vi "Measure vs B2Dv4.vi"() -> ()   [LabVIEW 2009]
doc: "This VI is an example operator panel.\n\nThe VI contains a table for the field values that may be configured manually, or loaded by checking the \"Prompt for File\" box. The data file should contain 3 columns of data, with each column delimited by a tab character.\n\nBefore the VI is executed, set the desired field units and coordinate system. Once the VI is started, follow the directions in the STATUS indicator to operate. Once a field value is achieved, it will be held indefinitely with no user intervention.\n\nThe present field is displayed in the selected units and coordinate system. The present field is queried once per second.\n\nIf a field point is specified that is outside the limits for the magnet, the VI will abort execution."
uses:
  <vilib>/Utility/file.llb/Read From Spreadsheet File (DBL).vi
panel:
  in  "Wait between \nVectors":bool
  in  "FieldRange":dbl=1.0
  in  "Change\nPID\n(DetermineSIMPID.vi)":bool
  in  "Wait between \nVectors (ms)":u32=3000
  in  "X Axis":enum16{"B", "phi"}(ring)
  in  "Y Axis":T1(ring)=enum."HP (V)"
  out "measured data":dbl[][](array[numeric])=[[1.000012086526958, 89.00072302371139, 0.0, 0.0, 0.0, 0.0, 0.0, 0.0, 0.0, 0.0, 20.70647, 3397102510.2661195], [0.9999822655427446, 89.00012016557346, 0.0, 0.0, 0.0, 0.0, 0.0, 0.0, 0.0, 0.0, 20.70772, 3397102511.0341196], [1.0000224339983579, 88.99958730013925, 0.0, 0.0, 0.0, 0.0, 0.0, 0.0, 0.0, 0.0, 20.70752, 3397102511.6071196], [1.0000220850061263, 89.00073301575388, 0.0, 0.0, 0.0, 0.0, 0.0, 0.0, 0.0, 0.0, 20.70772, 3397102512.18112], [0.9999922640200775, 89.00013016394165, 0.0, 0.0, 0.0, 0.0, 0.0, 0.0, 0.0, 0.0, 20.70689, 3397102512.7561197], [1.0000022624974407, 89.0001401621099, 0.0, 0.0, 0.0, 0.0, 0.0, 0.0, 0.0, 0.0, 20.70783, 3397102513.3311195], [1.0000122609748343, 89.00015016007822, 0.0, 0.0, 0.0, 0.0, 0.0, 0.0, 0.0, 0.0, 20.70835, 3397102513.9071198], [1.00000208804782, 89.00071303146908, 0.0, 0.0, 0.0, 0.0, 0.0, 0.0, 0.0, 0.0, 20.70845, 3397102514.4801197], [0.9999822655427446, 89.00012016557346, 0.0, 0.0, 0.0, 0.0, 0.0, 0.0, 0.0, 0.0, 20.70793, 3397102515.05712], [1.0000122609748343, 89.00015016007822, 0.0, 0.0, 0.0, 0.0, 0.0, 0.0, 0.0, 0.0, 20.70731, 3397102515.63012], [1.0000022624974407, 89.0001401621099, 0.0, 0.0, 0.0, 0.0, 0.0, 0.0, 0.0, 0.0, 20.70731, 3397102516.2041197], [0.9999822655427446, 89.00012016557346, 0.0, 0.0, 0.0, 0.0, 0.0, 0.0, 0.0, 0.0, 20.70606, 3397102516.7781196], [0.9999822655427446, 89.00012016557346, 0.0, 0.0, 0.0, 0.0, 0.0, 0.0, 0.0, 0.0, 20.70595, 3397102517.46612], [1.0000122609748343, 89.00015016007822, 0.0, 0.0, 0.0, 0.0, 0.0, 0.0, 0.0, 0.0, 20.70595, 3397102518.03712], [0.9999724416202679, 88.9995372806674, 0.0, 0.0, 0.0, 0.0, 0.0, 0.0, 0.0, 0.0, 20.70606, 3397102518.6131196]]
  out "XY Graph":T2(graph)={"measured data"=[1.000012086526958, 0.9999822655427446, 1.0000224339983579, 1.0000220850061263, 0.9999922640200775, 1.0000022624974407, 1.0000122609748343, 1.00000208804782, 0.9999822655427446, 1.0000122609748343, 1.0000022624974407, 0.9999822655427446, 0.9999822655427446, 1.0000122609748343, 0.9999724416202679], "measured data"=[20.70647, 20.70772, 20.70752, 20.70772, 20.70689, 20.70783, 20.70835, 20.70845, 20.70793, 20.70731, 20.70731, 20.70606, 20.70595, 20.70595, 20.70606]}
  in  "Notes:":string="Datum: 24.08.11, Uhrzeit: 16:26, T0.3K, PID LOOP: P -0.2 I 200 D off , PID Dämpfung: P off , Laser 25°, 20mA, AOM 10mA, Sweep 0.12T/min, Winkelsweep 90-0--280° bei 1 T,  Winkelschritt 0.4°, Position auf ansteigender Fringe" caption="Notizen:"
  out "Messfile Refnum":refnum<file>
  in  "Measurement File":path=path "D:/UserData/Matthias/Messungen/STO_LAOR103/110825/110824_R103_test.txt"
  in  "Sample name:":string="R103"
  in  "HP 1":bool=TRUE
  in  "GPIB HP":string="14"
  in  "LI 4":bool
  in  "GPIB L 4":string="8"
  in  "LI 3":bool
  in  "GPIB L 3":string="8"
  in  "LI 2":bool
  in  "GPIB L 2":string="8"
  in  "LI 1":bool
  in  "GPIB L 1":string="8"
  out "Number of lines":i32=2
  in  "Operation":u16(ring) items=["Stepwise", "Continous"]
  out "Ramp Rate along Vector (T/min)":dbl=0.17756501513530193 format="%.3f"
  out "Current Ramp Rate Z (T/min)":dbl=0.00639 format="%.3f"
  out "Current Ramp Rate Y (T/min)":dbl=0.17745 format="%.3f"
  in  "User defined Ramp Rate (T/min)":bool
  in  "User defined Ramp Rate (T/min)":dbl=0.12 format="%.3f"
  in  "Z-Axis Communications Config":T3={"GPIB address"=22, "GPIB bus"=1, "connection ID"=refnum, "IP"="111.111.111.1", "Active Comm Interface"=0, "Serial Port"="", "Programmer Type"=0} {"Programmer Type" items=["Model 430", "Model 420"]; "Active Comm Interface" items=["TCP/IP (Model 430 Only)", "RS232", "IEEE488"]}
  in  "Max Ramp Rate - Y Axis (A/s)":dbl=0.065 format="%.3f"
  in  "Max Ramp Rate - Z Axis (A/s)":dbl=0.203 format="%.3f"
  in  "Magnitude Limit (kG)":dbl=45.1 format="%.3f"
  in  "Y-Axis Communications Config":T3={"GPIB address"=22, "GPIB bus"=1, "connection ID"=refnum, "IP"="111.111.111.2", "Active Comm Interface"=0, "Serial Port"="", "Programmer Type"=0} {"Programmer Type" items=["Model 430", "Model 420"]; "Active Comm Interface" items=["TCP/IP (Model 430 Only)", "RS232", "IEEE488"]}
  out "Cartesian Display (T)":T4={"Y-Axis Field (T)"=0.01746, "Z-Axis Field (T)"=0.99986} {"Z-Axis Field (T)" format="%.3f"; "Y-Axis Field (T)" format="%.3f"}
  in  "Starting index":i32=1
  in  "Normal color":u32(colorbox)=11711154
  in  "Highlight color":u32(colorbox)=16711680
  in  "Prompt for File?":bool
  out "Continue Execution?":bool=TRUE
  out "error out":T5
  in  "error in":T5
  out "STATUS":string="All Programmers are PAUSED. Set Ramping Mode to NEXT VECTOR to continue."
  in  "Ramping Control":u16(ring)=3 items=["NEXT VECTOR", "RAMPING", "HOLDING", "PAUSE", "ZERO"]
  out "Cartesian Display (kG)":T6 {"Z-Axis Field (kG)" format="%.3f"; "Y-Axis Field (kG)" format="%.3f"}
  in  "Field Values":string[][](table)=[["1", "89"], ["", ""]]
  out "Switch Heaters":bool=TRUE
  out "Polar Display (T)":T7={"q (degrees)"=89.00013016394165, "Field Magnitude (T)"=0.9999922640200775} {"Field Magnitude (T)" format="%.3f"; "q (degrees)" format="%.3f"}
  out "Polar Display (kG)":T8 {"Field Magnitude (kG)" format="%.3f"; "q (degrees)" format="%.3f"}
  in  "Coordinate System":u16(ring)=1 items=["Cartesian", "Polar"]
  in  "Magnetic Field Units":u16(ring)=1 items=["kG", "Tesla"]
  # "Measurement Display"
  # "Measurement Settings"
  # "Magnet Settings"
  # "Max Ramp Rate z: 1.27 T/min\nMax Ramp Rate y: 0.17 T/min"
  # "Devices"
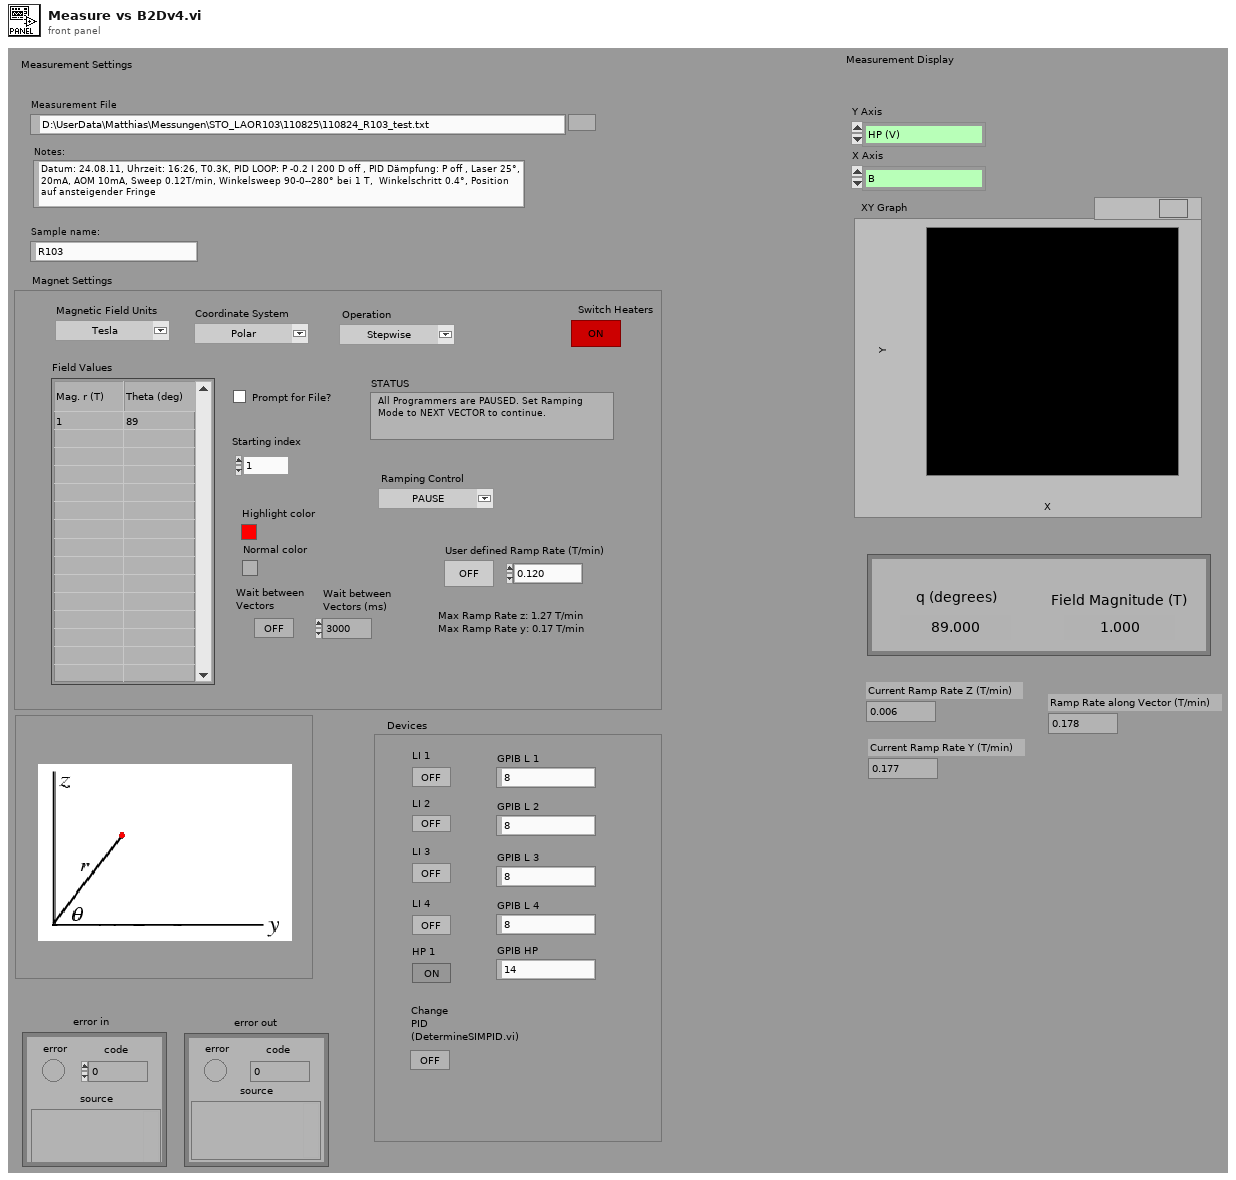
[diagram p1: front panel]
types:
  T1 = enum16{"B", "phi", "LI 1 Vx", "LI 1 phase", "LI 2 Vx", "LI 2 phase", "LI 3 Vx", "LI 3 phase", "LI 4 Vx", "LI 4 phase", "HP (V)"}
  T2 = cluster{"measured data":dbl[], "measured data":dbl[]}
  T3 = cluster{"GPIB address":i16, "GPIB bus":i16, "connection ID":refnum<k5>, "IP":string, "Active Comm Interface":u16, "Serial Port":refnum<visa-resource-name>, "Programmer Type":u16}
  T4 = cluster{"Y-Axis Field (T)":dbl, "Z-Axis Field (T)":dbl}
  T5 = cluster{"error":bool, "code":i32, "source":string}
  T6 = cluster{"Y-Axis Field (kG)":dbl, "Z-Axis Field (kG)":dbl}
  T7 = cluster{"q (degrees)":dbl, "Field Magnitude (T)":dbl}
  T8 = cluster{"q (degrees)":dbl, "Field Magnitude (kG)":dbl}
  T9 = enum16{"", "RAMPING", "HOLDING", "PAUSED", "MANUAL UP", "MANUAL DOWN", "ZEROING CURRENT", "QUENCH DETECTED", "HEATING SWITCH"}
  T10 = enum16{"", "RAMPING", "HOLDING", "PAUSED", "MANUAL UP", "MANUAL DOWN", "ZEROING CURRENT", "QUENCH DETECTED", "HEATING SWITCH", "AT ZER0", "COOLING SWITCH"}
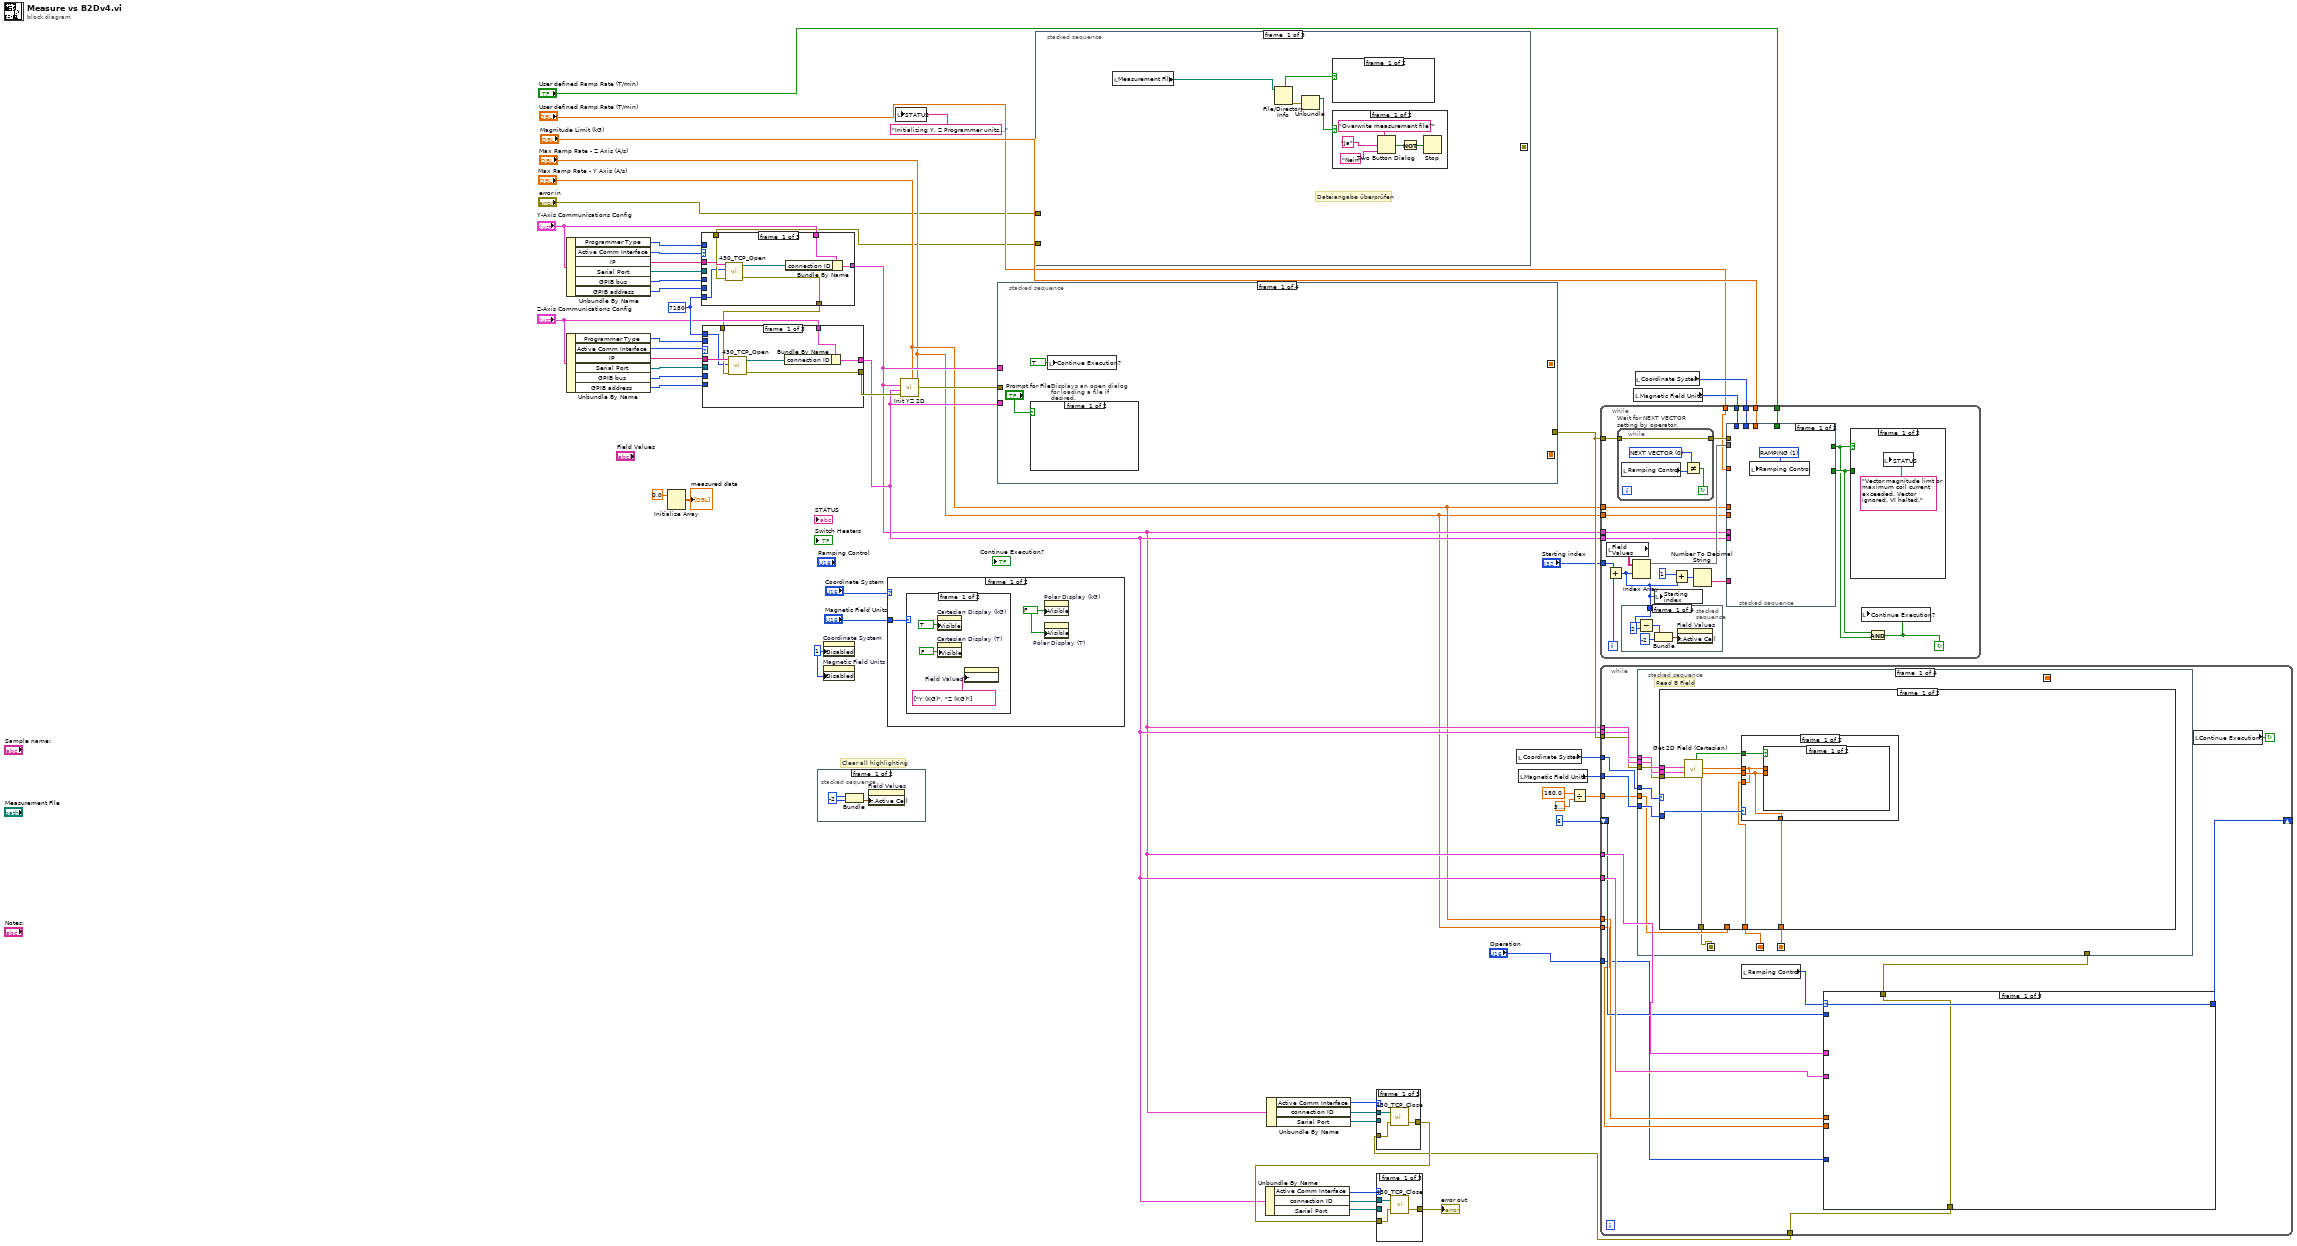
[diagram p0: block diagram]
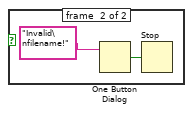
[diagram p3: hidden frame]
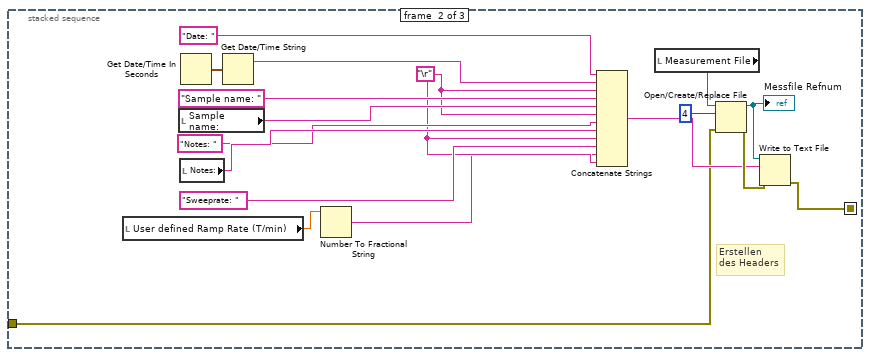
[diagram p4: hidden frame]
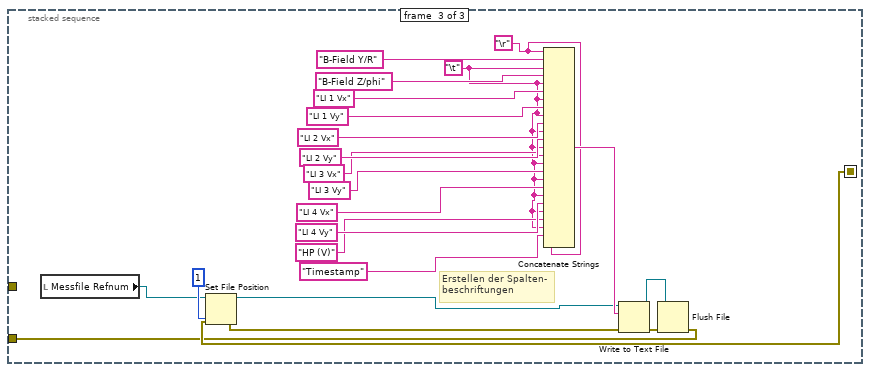
[diagram p5: hidden frame]
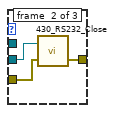
[diagram p6: hidden frame]
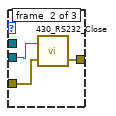
[diagram p8: hidden frame]
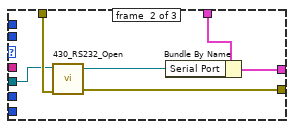
[diagram p10: hidden frame]
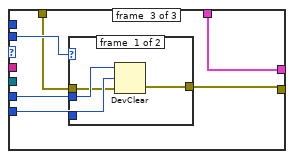
[diagram p11: hidden frame]
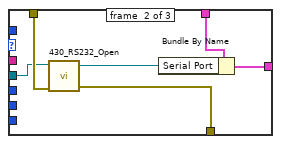
[diagram p13: hidden frame]
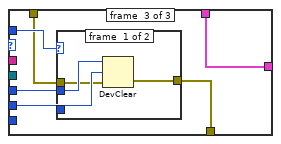
[diagram p14: hidden frame]
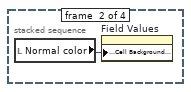
[diagram p16: hidden frame]
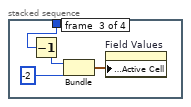
[diagram p17: hidden frame]
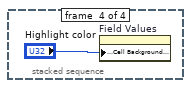
[diagram p18: hidden frame]
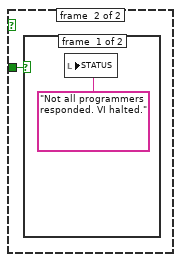
[diagram p19: hidden frame]
diagram:
  w38 = 7180 ("TCP Port")
  w51 = u8 1 ("Write Attribute")
  # "Clear all highlighting"
  n1 = Unbundle By Name("Z-Axis Communications Config") -> ("Programmer Type"=w14:u16, "Active Comm Interface"=w37:u16, "IP"=w34:string, "Serial Port"=w33:refnum<visa-resource-name>, "GPIB bus"=w13:i16, "GPIB address"=w12:i16)
  n2 = Unbundle By Name("Y-Axis Communications Config") -> ("Programmer Type"=w8:u16, "Active Comm Interface"=w36:u16, "IP"=w35:string, "Serial Port"=w32:refnum<visa-resource-name>, "GPIB bus"=w9:i16, "GPIB address"=w10:i16)
  n3 = Initialize Array(0.0 ("element")) -> (→"measured data":dbl[][])  [unwired: 2 in]
  n4 = stacked-sequence {
    frame #0 {
      w54 = -2
      n5 = Bundle(w54, w54) -> (w55:cluster{i32, i32})  [unwired: 1 in]
      n6 = property on="Field Values" class="Tbl (strict)"("Active Cell:Active Cell"=w55) -> ()  [unwired: 2 in, 2 out]
    }
    frame #1 {
      n7 = property on="Field Values" class="Tbl (strict)"("Active Cell:Cell Background Color"="Normal color") -> ()  [unwired: 2 in, 2 out]
    }
  }
  n8 = property on="Coordinate System" class="Ring (strict)"("Disabled"=w51) -> ()  [unwired: 2 in, 2 out]
  n9 = property on="Magnetic Field Units" class="Ring (strict)"("Disabled"=w51) -> ()  [unwired: 2 in, 2 out]
  n10 = case shown="0, Default" "Coordinate System" {
    tunnel: "Magnetic Field Units" -> [w58 w66]
    frame #0 {
      w57 = FALSE ("Write Attribute")
      (unwired) FALSE ("Write Attribute")
      (unwired) TRUE ("Write Attribute")
      n11 = case shown="1" w58 {
        frame #0 {
          n12 = property on="Cartesian Display (kG)" class="Cluster (strict)"("Visible"=TRUE ("Write Attribute")) -> ()  [unwired: 2 in, 2 out]
          n13 = property on="Cartesian Display (T)" class="Cluster (strict)"("Visible"=FALSE ("Write Attribute")) -> ()  [unwired: 2 in, 2 out]
          n14 = property on="Field Values" class="Tbl (strict)"("Column Header Strings[]"=string[] ["Y (KG)", "Z (KG)"] ("Write Attribute")) -> ()  [unwired: 2 in, 2 out]
        }
        frame #1 {
          n15 = property on="Cartesian Display (kG)" class="Cluster (strict)"("Visible"=FALSE ("Write Attribute")) -> ()  [unwired: 2 in, 2 out]
          n16 = property on="Cartesian Display (T)" class="Cluster (strict)"("Visible"=TRUE ("Write Attribute")) -> ()  [unwired: 2 in, 2 out]
          n17 = property on="Field Values" class="Tbl (strict)"("Column Header Strings[]"=string[] ["Y (T)", "Z (T)"] ("Write Attribute")) -> ()  [unwired: 2 in, 2 out]
        }
      }
      n18 = property on="Polar Display (kG)" class="Clust (strict)"("Visible"=w57) -> ()  [unwired: 2 in, 2 out]
      n19 = property on="Polar Display (T)" class="Clust (strict)"("Visible"=w57) -> ()  [unwired: 2 in, 2 out]
    }
    frame #1 {
      (unwired) FALSE ("Write Attribute")
      (unwired) TRUE ("Write Attribute")
      w65 = FALSE ("Write Attribute")
      n20 = case shown="1" w66 {
        frame #0 {
          n21 = property on="Polar Display (kG)" class="Clust (strict)"("Visible"=TRUE ("Write Attribute")) -> ()  [unwired: 2 in, 2 out]
          n22 = property on="Polar Display (T)" class="Clust (strict)"("Visible"=FALSE ("Write Attribute")) -> ()  [unwired: 2 in, 2 out]
          n23 = property on="Field Values" class="Tbl (strict)"("Column Header Strings[]"=string[] ["Mag. r (KG)", "Theta (deg)"] ("Write Attribute")) -> ()  [unwired: 2 in, 2 out]
        }
        frame #1 {
          n24 = property on="Polar Display (kG)" class="Clust (strict)"("Visible"=FALSE ("Write Attribute")) -> ()  [unwired: 2 in, 2 out]
          n25 = property on="Polar Display (T)" class="Clust (strict)"("Visible"=TRUE ("Write Attribute")) -> ()  [unwired: 2 in, 2 out]
          n26 = property on="Field Values" class="Tbl (strict)"("Column Header Strings[]"=string[] ["Mag. r (T)", "Theta (deg)"] ("Write Attribute")) -> ()  [unwired: 2 in, 2 out]
        }
      }
      n27 = property on="Cartesian Display (kG)" class="Cluster (strict)"("Visible"=w65) -> ()  [unwired: 2 in, 2 out]
      n28 = property on="Cartesian Display (T)" class="Cluster (strict)"("Visible"=w65) -> ()  [unwired: 2 in, 2 out]
    }
  }
  n29 = local write "STATUS"("Initializing Y, Z Programmer units..." ("STATUS")) -> ()
  n30 = stacked-sequence {
    seq-local: [_ w84 _] -> [_ _ w103]
    tunnel: "error in" -> [_ w85 _]
    tunnel: [_ _ w102] -> w3
    frame #0 {
      # "Dateiangabe überprüfen"
      n31 = local read "Measurement File"() -> (w76:path)
      n32 = File/Directory Info(path=w76) -> (directory=w74:bool, error out=w75:errorcluster)  [unwired: 1 in, 5 out]
      n33 = Unbundle(w75) -> ("status"=w73:bool)  [unwired: 2 out]
      n34 = case shown="False" w74 {
        frame #0 {
        }
        frame #1 {
          n35 = One Button Dialog(message="Invalid\nfilename!") -> (true=w82:bool)  [unwired: 1 in]
          n36 = Stop(stop? (T)=w82) -> ()
        }
      }
      n37 = case shown="False" w73 {
        frame #0 {
          n38 = Two Button Dialog(message="Overwrite measurement file?", 1:"Nein", 2:"Ja") -> (T button?=w78:bool)
          n39 = Not(x=w78) -> (.not. x?=w77:bool)
          n40 = Stop(stop? (T)=w77) -> ()
        }
        frame #1 {
        }
      }
    }
    frame #1 {
      w88 = "\r"
      # "Erstellen\ndes Headers"
      n41 = local read "User defined Ramp Rate (T/min)"() -> (w87:dbl)
      n42 = local read "Sample name:"() -> (w94:string)
      n43 = local read "Notes:"() -> (w96:string)
      n44 = Get Date/Time In Seconds() -> (seconds since 1Jan1904=w90:timestamp)
      n45 = Get Date/Time String(seconds (now)=w90) -> (date string=w92:string)  [unwired: 2 in, 1 out]
      n46 = Number To Fractional String(number=w87) -> (F-format string=w86:string)  [unwired: 3 in]
      n47 = Concatenate Strings("Date: ", w92, w88, "Sample name: ", w94, w88, "Notes: ", w96, w88, "Sweeprate: ", w86, w88) -> (w100:string)
      n48 = local read "Measurement File"() -> (w97:path)
      n49 = Open/Create/Replace File(file path (use dialog)=w97, error in=w85, operation (0:open)=4) -> (refnum out=w99:refnum<file>, error out=w101:errorcluster)  [unwired: 3 in, 1 out]
      "Messfile Refnum" <- w99
      n50 = Write to Text File(file (use dialog)=w99, text=w100, error in=w101) -> (error out=w84:errorcluster)  [unwired: 1 in, 2 out]
    }
    frame #2 {
      w106 = "\t"
      w104 = "\r"
      # "Erstellen der Spalten-\nbeschriftungen"
      n51 = local read "Messfile Refnum"() -> (w113:refnum<file>)
      n52 = Set File Position(refnum=w113, from (0:start)=1, error in=w103) -> (refnum out=w119:refnum<file>, error out=w121:errorcluster)  [unwired: 1 in]
      n53 = Concatenate Strings(w104, "B-Field Y/R", w106, "B-Field Z/phi", w106, "LI 1 Vx", w106, "LI 1 Vy", w106, "LI 2 Vx", w106, "LI 2 Vy", w106, "LI 3 Vx", w106, "LI 3 Vy", w106, "LI 4 Vx", w106, "LI 4 Vy", w106, "HP (V)", w106, "Timestamp", w104) -> (w120:string)
      n54 = Write to Text File(file (use dialog)=w119, text=w120, error in=w121) -> (refnum out=w123:refnum<file>, error out=w122:errorcluster)  [unwired: 1 in, 1 out]
      n55 = Flush File(refnum=w123, error in=w122) -> (error out=w102:errorcluster)  [unwired: 1 out]
    }
  }
  n56 = case shown="2" w36 {
    tunnel: w35 -> [w131 _ _]
    tunnel: w3 -> [w130 w137 w139]
    tunnel: "Y-Axis Communications Config" -> [w129 w132 w143]
    tunnel: [w127 w135 w143] -> w21
    tunnel: [w126 w136 w138] -> w11
    tunnel: w38 -> [w125 _ _]
    tunnel: w32 -> [_ w133 _]
    tunnel: w10 -> [_ _ w142]
    tunnel: w9 -> [_ _ w141]
    tunnel: w8 -> [_ _ w140]
    frame #0 {
      n57 = call <userlib>:"430_TCP_Open.vi"("IP Address"=w131, "TCP Port"=w125, "error in (no error)"=w130) -> ("connection ID"=w128:refnum<k5>, "error out"=w126:errorcluster)  [unwired: 3 in, 1 out]
      n58 = Bundle By Name(cluster=w129, "connection ID"=w128) -> (w127:T3)
    }
    frame #1 {
      n59 = call <userlib>:"430_RS232_Open.vi"("VISA resource name"=w133, "error in (no error)"=w137) -> ("VISA resource name out"=w134:refnum<visa-resource-name>, "error out"=w136:errorcluster)  [unwired: 5 in]
      n60 = Bundle By Name(cluster=w132, "Serial Port"=w134) -> (w135:T3)
    }
    frame #2 {
      n61 = case shown="0, Default" w140 {
        tunnel: w141 -> [w147 _]
        tunnel: w142 -> [w146 _]
        tunnel: w139 -> [w145 w148]
        tunnel: [w144 w148] -> w138
        frame #0 {
          n62 = DevClear(2:w145, 3:w146, 4:w147) -> (0:w144:errorcluster)  [unwired: 1 out]
        }
        frame #1 {
        }
      }
    }
  }
  n63 = case shown="2" w37 {
    tunnel: w34 -> [w155 _ _]
    tunnel: w11 -> [w154 w161 w163]
    tunnel: [w153 w160 w162] -> w31
    tunnel: "Z-Axis Communications Config" -> [w152 w158 w167]
    tunnel: [w150 w159 w167] -> w22
    tunnel: w38 -> [w149 _ _]
    tunnel: w33 -> [_ w156 _]
    tunnel: w14 -> [_ _ w166]
    tunnel: w13 -> [_ _ w165]
    tunnel: w12 -> [_ _ w164]
    frame #0 {
      n64 = call <userlib>:"430_TCP_Open.vi"("IP Address"=w155, "TCP Port"=w149, "error in (no error)"=w154) -> ("connection ID"=w151:refnum<k5>, "error out"=w153:errorcluster)  [unwired: 3 in, 1 out]
      n65 = Bundle By Name(cluster=w152, "connection ID"=w151) -> (w150:T3)
    }
    frame #1 {
      n66 = call <userlib>:"430_RS232_Open.vi"("VISA resource name"=w156, "error in (no error)"=w161) -> ("VISA resource name out"=w157:refnum<visa-resource-name>, "error out"=w160:errorcluster)  [unwired: 5 in]
      n67 = Bundle By Name(cluster=w158, "Serial Port"=w157) -> (w159:T3)
    }
    frame #2 {
      n68 = case shown="0, Default" w166 {
        tunnel: w165 -> [w171 _]
        tunnel: w164 -> [w170 _]
        tunnel: w163 -> [w169 w172]
        tunnel: [w168 w172] -> w162
        frame #0 {
          n69 = DevClear(2:w169, 3:w170, 4:w171) -> (0:w168:errorcluster)  [unwired: 1 out]
        }
        frame #1 {
        }
      }
    }
  }
  n70 = call <userlib>:"Init YZ 2D.vi"("Max Ramp Rate Z-axis"="Max Ramp Rate - Z Axis (A/s)", "Max Ramp Rate Y-axis"="Max Ramp Rate - Y Axis (A/s)", "error in"=w31, "Z-Axis Communications Config"=w22, "Y-Axis Communications Config"=w21) -> ("error out"=w49:T5)  [unwired: 5 in]
  n71 = stacked-sequence {
    seq-local: [_ w180 _ _] -> [_ _ w227 _]
    seq-local: [_ w179 _ _] -> [_ _ w226 _]
    tunnel: w22 -> [_ w182 _ _]
    tunnel: w49 -> [_ w183 _ _]
    tunnel: [_ w178 _ _] -> w45
    tunnel: w21 -> [_ w181 _ _]
    frame #0 {
      n72 = case "Displays an open dialog for loading a file if desired." shown="True" "Prompt for File?" {
        frame #0 {
        }
        frame #1 {
          n73 = call-poly <vilib>:"Read From Spreadsheet File.vi"() -> ("all rows"=w177:dbl[][])  [unwired: 7 in, 4 out]
          n74 = Number To Fractional String(number=w177, precision (6)=i16 4) -> (F-format string=w176:string[][])  [unwired: 2 in]
          n75 = local write "Field Values"(w176) -> ()
        }
      }
      n76 = local write "Continue Execution?"(TRUE ("Continue Execution?")) -> ()
    }
    frame #1 {
      w191 = u16 3 items=["NEXT VECTOR", "RAMPING", "HOLDING", "PAUSE", "ZERO"] ("Ramping Control")
      n77 = call <userlib>:"Get Switch Present.vi"("error in"=w183, "Communications Config"=w181) -> ("error out"=w187:T5, "Switch Present?"=w188:bool)
      n78 = case shown="True" w188 {
        tunnel: w187 -> [w209 w218]
        tunnel: w181 -> [_ w211]
        tunnel: [0.0 w215] -> w179
        tunnel: [w209 w217] -> w186
        frame #0 {
        }
        frame #1 {
          n79 = call <userlib>:"Get Switch Heater Time.vi"("error in"=w218, "Communications Config"=w211) -> ("error out"=w214:T5, "Switch Heating Time (secs)"=w216:dbl)
          n80 = call <userlib>:"Get Switch Heater.vi"("error in"=w214, "Communications Config"=w211) -> ("error out"=w213:T5, "Switch Heater Indicator"=w212:bool)
          n81 = case shown="False" w212 {
            tunnel: [w223 w224] -> w217
            tunnel: w216 -> [w221 _]
            tunnel: [w221 0.0] -> w215
            tunnel: w213 -> [w219 w224]
            tunnel: w211 -> [w220 _]
            frame #0 {
              n82 = call <userlib>:"Set Switch Heater.vi"("error in"=w219, "Switch Heater Control"=TRUE, "Communications Config"=w220) -> ("error out"=w223:T5)
            }
            frame #1 {
            }
          }
        }
      }
      n83 = call <userlib>:"Get Switch Present.vi"("error in"=w186, "Communications Config"=w182) -> ("error out"=w184:T5, "Switch Present?"=w185:bool)
      n84 = case shown="True" w185 {
        tunnel: w184 -> [w192 w201]
        tunnel: w182 -> [_ w194]
        tunnel: [0.0 w198] -> w180
        tunnel: [w192 w200] -> w178
        frame #0 {
        }
        frame #1 {
          n85 = call <userlib>:"Get Switch Heater Time.vi"("error in"=w201, "Communications Config"=w194) -> ("error out"=w197:T5, "Switch Heating Time (secs)"=w199:dbl)
          n86 = call <userlib>:"Get Switch Heater.vi"("error in"=w197, "Communications Config"=w194) -> ("error out"=w196:T5, "Switch Heater Indicator"=w195:bool)
          n87 = case shown="False" w195 {
            tunnel: [w202 w207] -> w200
            tunnel: w199 -> [w205 _]
            tunnel: [w205 0.0] -> w198
            tunnel: w196 -> [w203 w207]
            tunnel: w194 -> [w204 _]
            frame #0 {
              n88 = call <userlib>:"Set Switch Heater.vi"("error in"=w203, "Switch Heater Control"=TRUE, "Communications Config"=w204) -> ("error out"=w202:T5)
            }
            frame #1 {
            }
          }
        }
      }
      n89 = local write "Ramping Control"(w191) -> ()
      n90 = local write "Switch Heaters"(TRUE ("Switch Heater Control")) -> ()
      n91 = property on="Switch Heaters" class="Boolean (strict)"("Disabled"=u8 1 ("Write Attribute")) -> ()  [unwired: 2 in, 2 out]
    }
    frame #2 {
      n92 = Max & Min(x=w227, y=w226) -> (max(x,y)=w228:dbl)  [unwired: 1 out]
      n93 = local write "STATUS"("Heating switches..." ("STATUS")) -> ()
      n94 = Add(x=w228, y=2) -> (x+y=w232:dbl)
      n95 = property on="Ramping Control" class="Ring (strict)"("Disabled"=u8 1 ("Write Attribute")) -> ()  [unwired: 2 in, 2 out]
      n96 = Multiply(x=w232, y=1000) -> (x*y=w231:dbl)
      n97 = Wait (ms)(milliseconds to wait=w231) -> ()  [unwired: 1 out]
    }
    frame #3 {
      n98 = property on="Ramping Control" class="Ring (strict)"("Disabled"=u8 0 ("Write Attribute")) -> ()  [unwired: 2 in, 2 out]
      n99 = local write "STATUS"("Ready to ramp to first vector. Set Ramping Mode to NEXT VECTOR to begin." ("STATUS")) -> ()
      n100 = local read "Field Values"() -> (w237:string[][])
      n101 = Array Size(array=w237) -> (size(s)=w236:i32[])
      n102 = Index Array(array=w236, index=0) -> (element=→"Number of lines":i32)
    }
  }
  n103 = Unbundle By Name(w22) -> ("Active Comm Interface"=w28:u16, "connection ID"=w27:refnum<k5>, "Serial Port"=w26:refnum<visa-resource-name>)
  n104 = Unbundle By Name(w21) -> ("Active Comm Interface"=w29:u16, "connection ID"=w25:refnum<k5>, "Serial Port"=w24:refnum<visa-resource-name>)
  n105 = local read "Coordinate System"() -> (w46:u16)
  n106 = local read "Magnetic Field Units"() -> (w44:u16)
  n107 = Divide(x=180.0, y=3.141592653589793) -> (x/y=w41:dbl)
  n108 = while {
    shift-left: u16 6 ("Ramping Control") -> [w245]
    shift-right: [w246] -> _
    tunnel: [w248] -> w23
    tunnel: w22 -> [w249]
    tunnel: w21 -> [w250]
    tunnel: w41 -> [w252]
    tunnel: w44 -> [w253]
    tunnel: w45 -> [w254]
    tunnel: w22 -> [w255]
    tunnel: w21 -> [w256]
    tunnel: w46 -> [w257]
    tunnel: "Max Ramp Rate - Y Axis (A/s)" -> [w244]
    tunnel: "Max Ramp Rate - Z Axis (A/s)" -> [w243]
    tunnel: "Operation" -> [w242]
    stop <- w247 continue-if-true
    n109 = stacked-sequence {
      seq-local: [w260 _ _ _] -> [_ _ w360 _]
      seq-local: [w259 _ _ _] -> [_ w329 w357 _]
      seq-local: [w258 _ _ _] -> [_ _ w358 _]
      seq-local: [_ _ w344 _] -> [_ _ _ w428]
      tunnel: w257 -> [w266 _ _ w426]
      tunnel: w256 -> [w265 _ _ _]
      tunnel: w255 -> [w264 _ _ _]
      tunnel: w254 -> [w263 _ _ _]
      tunnel: w253 -> [w262 _ _ _]
      tunnel: w252 -> [w261 _ _ _]
      tunnel: [_ _ w359 _] -> w241
      frame #0 {
        # "Read B Field"
        n110 = case shown="0, Default" w266 {
          tunnel: w265 -> [w276 w299]
          tunnel: w264 -> [w275 w298]
          tunnel: w263 -> [w274 w297]
          tunnel: w262 -> [w273 w296]
          tunnel: w261 -> [_ w295]
          tunnel: [w269 w294] -> w260
          tunnel: [w268 w292] -> w259
          tunnel: [w267 w293] -> w258
          frame #0 {
            n111 = call <userlib>:"Get 2D Field (Cartesian).vi"("Y-Axis Communications Config"=w276, "Z-Axis Communications Config"=w275, "error in"=w274) -> ("All Instruments Responded?"=w270:bool, "Y-Axis Field (kG)"=w272:dbl, "Z-Axis Field (kG)"=w271:dbl, "error out"=w269:T5)  [unwired: 2 in]
            n112 = case shown="0, Default" w273 {
              tunnel: w272 -> [w277 w285]
              tunnel: w271 -> [w278 w286]
              tunnel: w270 -> [w279 w288]
              tunnel: [w278 w284] -> w268
              tunnel: [w277 w283] -> w267
              frame #0 {
                n113 = case shown="True" w279 {
                  tunnel: w277 -> [_ w281]
                  tunnel: w278 -> [_ w280]
                  frame #0 {
                  }
                  frame #1 {
                    n114 = Bundle("Y-Axis Field (kG)"=w281, "Z-Axis Field (kG)"=w280) -> (→"Cartesian Display (kG)":T6)  [unwired: 1 in]
                  }
                }
              }
              frame #1 {
                w287 = 0.1 ("y")
                n115 = Multiply(x=w285, y=w287) -> (x*y=w283:dbl)
                n116 = Multiply(x=w286, y=w287) -> (x*y=w284:dbl)
                n117 = case shown="True" w288 {
                  tunnel: w283 -> [_ w291]
                  tunnel: w284 -> [_ w290]
                  frame #0 {
                  }
                  frame #1 {
                    n118 = Bundle(w291, w290) -> (→"Cartesian Display (T)":cluster{dbl, dbl})  [unwired: 1 in]
                  }
                }
              }
            }
          }
          frame #1 {
            n119 = stacked-sequence {
              tunnel: w299 -> [w310]
              tunnel: w298 -> [w309]
              tunnel: w297 -> [w308]
              tunnel: w296 -> [w307]
              tunnel: w295 -> [w304]
              tunnel: [w302] -> w294
              tunnel: [w301] -> w292
              tunnel: [w300] -> w293
              frame #0 {
                # "Field"
                n120 = call <userlib>:"Get 2D Field (Polar).vi"("Y-Axis Communications Config"=w310, "Z-Axis Communications Config"=w309, "error in"=w308) -> ("All Instruments Responded?"=w303:bool, "Radial (r) Field (kG)"=w306:dbl, "q (radians)"=w305:dbl, "error out"=w302:T5)  [unwired: 2 in]
                n121 = case shown="1" w307 {
                  tunnel: w306 -> [w312 w324]
                  tunnel: w305 -> [w314 w323]
                  tunnel: w304 -> [w313 w322]
                  tunnel: w303 -> [w315 w321]
                  tunnel: [w312 w319] -> w301
                  tunnel: [w311 w320] -> w300
                  frame #0 {
                    n122 = Multiply(x=w314, y=w313) -> (x*y=w311:dbl)
                    n123 = case shown="True" w315 {
                      tunnel: w312 -> [_ w316]
                      tunnel: w311 -> [_ w317]
                      frame #0 {
                      }
                      frame #1 {
                        n124 = Bundle(w317, "Radial (r) Field (kG)"=w316) -> (→"Polar Display (kG)":cluster{dbl, "Radial (r) Field (kG)":dbl})  [unwired: 1 in]
                      }
                    }
                  }
                  frame #1 {
                    n125 = Multiply(x=w324, y=0.1) -> (x*y=w320:dbl)
                    n126 = Multiply(x=w323, y=w322) -> (x*y=w319:dbl)
                    n127 = case shown="True" w321 {
                      tunnel: w320 -> [_ w326]
                      tunnel: w319 -> [_ w327]
                      frame #0 {
                      }
                      frame #1 {
                        n128 = Bundle(w327, w326) -> (→"Polar Display (T)":cluster{dbl, dbl})  [unwired: 1 in]
                      }
                    }
                  }
                }
              }
            }
          }
        }
      }
      frame #1 {
        # "Change PID"
        n129 = case shown="True" "Change\nPID\n(DetermineSIMPID.vi)" {
          tunnel: w329 -> [_ w334]
          frame #0 {
          }
          frame #1 {
            # "z Field Value"
            n130 = call "CheckFieldRange.vi"("Field Value"=w334) -> ("Field Range"=w331:dbl)  [unwired: 10 in]
            n131 = Equal?(x="FieldRange", y=w331) -> (x = y?=w333:bool)
            n132 = case shown="False" w333 {
              tunnel: w331 -> [w339 w340]
              frame #0 {
                n133 = local write "FieldRange"(w339) -> ()
                n134 = call "DetermineSIMPID.vi"("Field Range"=w339) -> ("D"=w337:string, "P"=w338:string)  [unwired: 7 in, 2 out]
                n135 = call "SIM960ChangeP.vi"("New D Value"=w337, "New P Value"=w338, "Port Num- PID"="1", "GPIB-Adress"="2") -> ()  [unwired: 8 in]
              }
              frame #1 {
                n136 = local write "FieldRange"(w340) -> ()
              }
            }
          }
        }
      }
      frame #2 {
        w343 = u16 2 items=["NEXT VECTOR", "RAMPING", "HOLDING", "PAUSE", "ZERO"] ("Ramping Control")
        # "Zeile in Datei schreiben"
        # "Read and Save Devices"
        n137 = stacked-sequence {
          tunnel: [w372 _ _ _ _ _] -> w356
          tunnel: [w371 _ _ _ _ _] -> w355
          tunnel: [_ w385 _ _ _ _] -> w352
          tunnel: [_ w383 _ _ _ _] -> w351
          tunnel: [_ _ w395 _ _ _] -> w350
          tunnel: [_ _ w394 _ _ _] -> w349
          tunnel: [_ _ _ w406 _ _] -> w348
          tunnel: [_ _ _ w405 _ _] -> w347
          tunnel: [_ _ _ _ w416 _] -> w346
          tunnel: [_ _ _ _ _ w422] -> w345
          frame #0 {
            n138 = case shown="True" "LI 1" {
              tunnel: ["0" ("Antwort2") w379] -> w374
              tunnel: ["0" ("Antwort1") w378] -> w373
              frame #0 {
              }
              frame #1 {
                n139 = call "LI-Ansteuerung.vi"("Frage2"="OUTP? 4", "Frage1"="OUTP? 1", "address string"="GPIB L 1") -> ("Antwort2"=w379:string, "Antwort1"=w378:string)
              }
            }
            n140 = Fract/Exp String To Number(string=w374) -> (number=w371:dbl)  [unwired: 3 in, 1 out]
            n141 = Fract/Exp String To Number(string=w373) -> (number=w372:dbl)  [unwired: 3 in, 1 out]
          }
          frame #1 {
            n142 = case shown="False" "LI 2" {
              tunnel: [w388 w390] -> w384
              tunnel: [w388 w389] -> w386
              frame #0 {
                w388 = "0" ("Antwort1")
              }
              frame #1 {
                n143 = call "LI-Ansteuerung.vi"("Frage2"="OUTP? 4", "Frage1"="OUTP? 1", "address string"="GPIB L 2") -> ("Antwort2"=w390:string, "Antwort1"=w389:string)
              }
            }
            n144 = Fract/Exp String To Number(string=w384) -> (number=w383:dbl)  [unwired: 3 in, 1 out]
            n145 = Fract/Exp String To Number(string=w386) -> (number=w385:dbl)  [unwired: 3 in, 1 out]
          }
          frame #2 {
            n146 = case shown="False" "LI 3" {
              tunnel: [w399 w401] -> w396
              tunnel: [w399 w400] -> w397
              frame #0 {
                w399 = "0" ("Antwort1")
              }
              frame #1 {
                n147 = call "LI-Ansteuerung.vi"("Frage2"="OUTP? 4", "Frage1"="OUTP? 1", "address string"="GPIB L 3") -> ("Antwort2"=w401:string, "Antwort1"=w400:string)
              }
            }
            n148 = Fract/Exp String To Number(string=w397) -> (number=w395:dbl)  [unwired: 3 in, 1 out]
            n149 = Fract/Exp String To Number(string=w396) -> (number=w394:dbl)  [unwired: 3 in, 1 out]
          }
          frame #3 {
            n150 = case shown="True" "LI 4" {
              tunnel: [w410 w412] -> w407
              tunnel: [w410 w411] -> w408
              frame #0 {
                w410 = "0" ("Antwort1")
              }
              frame #1 {
                n151 = call "LI-Ansteuerung.vi"("Frage2"="OUTP? 4", "Frage1"="OUTP? 1", "address string"="GPIB L 4") -> ("Antwort2"=w412:string, "Antwort1"=w411:string)
              }
            }
            n152 = Fract/Exp String To Number(string=w407) -> (number=w405:dbl)  [unwired: 3 in, 1 out]
            n153 = Fract/Exp String To Number(string=w408) -> (number=w406:dbl)  [unwired: 3 in, 1 out]
          }
          frame #4 {
            n154 = case shown="True" "HP 1" {
              tunnel: [0.0 ("Voltage") w420] -> w416
              frame #0 {
              }
              frame #1 {
                n155 = call "HP-ReadVoltagev2.vi"("String"="meas:volt:dc? 200,0.001", "HP-Mulitmeter\nGPIB Address"="GPIB HP") -> ("Voltage"=w420:dbl)  [unwired: 9 in]
              }
            }
          }
          frame #5 {
            n156 = Get Date/Time In Seconds() -> (seconds since 1Jan1904=w423:timestamp)
            n157 = To Double Precision Float(number=w423) -> (double precision float=w422:dbl)
          }
        }
        n158 = local read "Ramping Control"() -> (w342:u16)
        n159 = Build Array(w358, w357, w356, w355, w352, w351, w349, w350, w348, w347, w346, w345) -> (w344:dbl[])
        n160 = Array To Spreadsheet String(array=w344, 3:"%f" ("format string")) -> (spreadsheet string=w354:string)  [unwired: 1 in]
        n161 = Equal?(x=w342, y=w343) -> (x = y?=w341:bool)
        n162 = case shown="False" w341 {
          tunnel: w360 -> [w369 w370]
          tunnel: [w368 w370] -> w359
          tunnel: w354 -> [w367 _]
          frame #0 {
            n163 = local read "Messfile Refnum"() -> (w361:refnum<file>)
            n164 = Set File Position(refnum=w361, from (0:start)=1, error in=w369) -> (refnum out=w363:refnum<file>, error out=w364:errorcluster)  [unwired: 1 in]
            n165 = Write to Text File(file (use dialog)=w363, text=w367, error in=w364) -> (refnum out=w366:refnum<file>, error out=w365:errorcluster)  [unwired: 1 in, 1 out]
            n166 = Flush File(refnum=w366, error in=w365) -> (error out=w368:errorcluster)  [unwired: 1 out]
          }
          frame #1 {
          }
        }
      }
      frame #3 {
        n167 = local read "measured data"() -> (w429:dbl[][])
        n168 = Insert Into Array(array=w429, new element=w428) -> (w427:dbl[][])  [unwired: 2 in]
        n169 = case shown="1" w426 {
          tunnel: w427 -> [w445 w459]
          tunnel: "Y Axis" -> [w447 w458]
          tunnel: "X Axis" -> [w435 w457]
          frame #0 {
            n170 = Index Array(array=w445, index (col)=1 ("disabled index (col)")) -> (element=w440:dbl[])  [unwired: 1 in]
            n171 = Index Array(array=w445, index (col)=0 ("disabled index (col)")) -> (element=w439:dbl[])  [unwired: 1 in]
            n172 = Square(x=w440) -> (x^2=w442:dbl[])
            n173 = Square(x=w439) -> (x^2=w443:dbl[])
            n174 = Index Array(array=w445, index (col)=w447) -> (element=w434:dbl[])  [unwired: 1 in]
            n175 = Divide(x=w440, y=w439) -> (x/y=w431:dbl[])
            n176 = Add(x=w443, y=w442) -> (x+y=w441:dbl[])
            n177 = Inverse Tangent(1:w431) -> (0:w430:dbl[])
            n178 = Square Root(x=w441) -> (sqrt(x)=w432:dbl[])
            n179 = Divide(x=w430, y=3.141592653589793) -> (x/y=w437:dbl[])
            n180 = Multiply(x=w437, y=180) -> (x*y=w433:dbl[])
            n181 = case shown="\"B\", Default" w435 {
              tunnel: w434 -> [w450 w453]
              tunnel: w433 -> [_ w452]
              tunnel: w432 -> [w449 _]
              frame #0 {
                n182 = Bundle(w449, "measured data"=w450) -> (w448:cluster{dbl[], "measured data":dbl[]})  [unwired: 1 in]
                n183 = local write "XY Graph"(w448) -> ()
              }
              frame #1 {
                n184 = Bundle(w452, "measured data"=w453) -> (w451:cluster{dbl[], "measured data":dbl[]})  [unwired: 1 in]
                n185 = local write "XY Graph"(w451) -> ()
              }
            }
          }
          frame #1 {
            n186 = Index Array(array=w459, index (col)=w457) -> (element=w456:dbl[])  [unwired: 1 in]
            n187 = Index Array(array=w459, index (col)=w458) -> (element=w455:dbl[])  [unwired: 1 in]
            n188 = Bundle("measured data"=w456, "measured data"=w455) -> (w454:T2)  [unwired: 1 in]
            n189 = local write "XY Graph"(w454) -> ()
          }
        }
        n190 = local write "measured data"(w427) -> ()
      }
    }
    n191 = local read "Ramping Control"() -> (w251:u16)
    n192 = case shown="4" w251 {
      selector: w251 -> [w461 w476 w499 w503 w518]
      tunnel: w250 -> [_ w479 _ w506 w523]
      tunnel: w249 -> [_ w478 _ w505 w522]
      tunnel: [w460 w477 w498 w504 w521] -> w248
      tunnel: [w461 w476 w499 w503 w518] -> w246
      tunnel: w245 -> [_ _ _ w502 w520]
      tunnel: w244 -> [_ _ _ _ w517]
      tunnel: w243 -> [_ _ _ _ w516]
      tunnel: w242 -> [_ w468 _ _ _]
      tunnel: w241 -> [w460 w464 w498 w500 w515]
      frame #0 {
      }
      frame #1 {
        w471 = T9."HOLDING" ("y")
        n193 = local read "Number of lines"() -> (w465:i32)
        n194 = local read "Starting index"() -> (w467:i32)
        n195 = call <userlib>:"Get Ramping Mode.vi"("Communications Config"=w479, "error in"=w464) -> ("Ramping Mode"=w474:T10, "error out"=w475:T5)  [unwired: 1 out]
        n196 = call <userlib>:"Get Ramping Mode.vi"("Communications Config"=w478, "error in"=w475) -> ("Ramping Mode"=w473:T10, "error out"=w477:T5)  [unwired: 1 out]
        n197 = Less?(x=w467, y=w465) -> (x < y?=w466:bool)
        n198 = Equal?(x=w474, y=w471) -> (x = y?=w470:bool)
        n199 = Equal?(x=w473, y=w471) -> (x = y?=w469:bool)
        n200 = Compound Arithmetic op=AND(w470, w469) -> (w472:bool)
        n201 = case shown="True" w472 {
          tunnel: w468 -> [_ w483]
          tunnel: w466 -> [_ w482]
          tunnel: "Wait between \nVectors (ms)" -> [_ w481]
          tunnel: "Wait between \nVectors" -> [_ w480]
          frame #0 {
          }
          frame #1 {
            n202 = case shown="0, Default" w483 {
              tunnel: w482 -> [_ w488]
              tunnel: w481 -> [_ w487]
              tunnel: w480 -> [_ w486]
              frame #0 {
                w485 = u16 2 items=["NEXT VECTOR", "RAMPING", "HOLDING", "PAUSE", "ZERO"] ("Ramping Control")
                n203 = local write "STATUS"("Holding at current vector. Set Ramping Mode to NEXT VECTOR to continue." ("STATUS")) -> ()
                n204 = local write "Ramping Control"(w485) -> ()
              }
              frame #1 {
                # "Go to NEXT VECTOR automatically"
                n205 = case shown="True" w488 {
                  tunnel: w487 -> [_ w492]
                  tunnel: w486 -> [_ w491]
                  frame #0 {
                    w490 = u16 2 items=["NEXT VECTOR", "RAMPING", "HOLDING", "PAUSE", "ZERO"] ("Ramping Control")
                    n206 = local write "STATUS"("Holding at current vector. Set Ramping Mode to NEXT VECTOR to continue." ("STATUS")) -> ()
                    n207 = local write "Ramping Control"(w490) -> ()
                  }
                  frame #1 {
                    n208 = stacked-sequence {
                      tunnel: w492 -> [w494 _]
                      tunnel: w491 -> [w493 _]
                      frame #0 {
                        n209 = case shown="True" w493 {
                          tunnel: w494 -> [_ w495]
                          frame #0 {
                          }
                          frame #1 {
                            n210 = Wait (ms)(milliseconds to wait=w495) -> ()  [unwired: 1 out]
                          }
                        }
                      }
                      frame #1 {
                        w497 = u16 0 items=["NEXT VECTOR", "RAMPING", "HOLDING", "PAUSE", "ZERO"] ("Ramping Control")
                        n211 = local write "Ramping Control"(w497) -> ()
                        n212 = local write "STATUS"("Go to NEXT VECTOR" ("STATUS")) -> ()
                      }
                    }
                  }
                }
              }
            }
          }
        }
      }
      frame #2 {
      }
      frame #3 {
        n213 = Not Equal?(x=w503, y=w502) -> (x != y?=w501:bool)
        n214 = case shown="False" w501 {
          tunnel: w506 -> [_ w514]
          tunnel: w505 -> [_ w513]
          tunnel: [w507 w511] -> w504
          tunnel: w500 -> [w507 w508]
          frame #0 {
          }
          frame #1 {
            w509 = u16 1 items=["RAMP", "PAUSE", "MANUAL UP", "MANUAL DOWN", "ZERO"] ("Ramping Mode")
            n215 = call <userlib>:"Set Ramping Mode.vi"("error in"=w508, "Ramping Mode"=w509, "Communications Config"=w514) -> ("error out"=w512:T5)
            n216 = call <userlib>:"Set Ramping Mode.vi"("error in"=w512, "Ramping Mode"=w509, "Communications Config"=w513) -> ("error out"=w511:T5)
            n217 = local write "STATUS"("All Programmers are PAUSED. Set Ramping Mode to NEXT VECTOR to continue." ("STATUS")) -> ()
          }
        }
      }
      frame #4 {
        n218 = Not Equal?(x=w518, y=w520) -> (x != y?=w519:bool)
        n219 = case shown="False" w519 {
          tunnel: w523 -> [_ w532]
          tunnel: w522 -> [_ w531]
          tunnel: [w524 w527] -> w521
          tunnel: w517 -> [_ w530]
          tunnel: w516 -> [_ w529]
          tunnel: w515 -> [w524 w525]
          frame #0 {
          }
          frame #1 {
            w526 = u16 4 items=["RAMP", "PAUSE", "MANUAL UP", "MANUAL DOWN", "ZERO"] ("Ramping Mode")
            n220 = local write "STATUS"("Zeroing vector." ("STATUS")) -> ()
            n221 = call <userlib>:"Set Ramping Mode.vi"("error in"=w525, "Ramping Mode"=w526, "Communications Config"=w532) -> ("error out"=w535:T5)
            n222 = call <userlib>:"Set Ramping Mode.vi"("error in"=w535, "Ramping Mode"=w526, "Communications Config"=w531) -> ("error out"=w528:T5)
            n223 = call <userlib>:"Set Current Ramp Rate.vi"("Communications Config"=w532, "Ramp Rate (A/sec)"=w530, "error in"=w528) -> ("error out"=w533:T5)  [unwired: 2 in]
            n224 = call <userlib>:"Set Current Ramp Rate.vi"("Communications Config"=w531, "Ramp Rate (A/sec)"=w529, "error in"=w533) -> ("error out"=w527:T5)  [unwired: 2 in]
          }
        }
      }
    }
    n225 = local read "Continue Execution?"() -> (w247:bool)
  }
  n226 = case shown="0, Default" w29 {
    tunnel: w25 -> [w538 _ _]
    tunnel: w23 -> [w537 w541 w542]
    tunnel: [w536 w540 w542] -> w30
    tunnel: w24 -> [_ w539 _]
    frame #0 {
      n227 = call <userlib>:"430_TCP_Close.vi"("error in (no error)"=w537, "connection ID"=w538) -> ("error out"=w536:errorcluster)  [unwired: 1 out]
    }
    frame #1 {
      n228 = call <userlib>:"430_RS232_Close.vi"("error in (no error)"=w541, "VISA resource name"=w539) -> ("error out"=w540:errorcluster)  [unwired: 1 in]
    }
    frame #2 {
    }
  }
  n229 = case shown="0, Default" w28 {
    tunnel: w27 -> [w545 _ _]
    tunnel: w30 -> [w544 w548 w549]
    tunnel: [w543 w547 w549] -> w20
    tunnel: w26 -> [_ w546 _]
    frame #0 {
      n230 = call <userlib>:"430_TCP_Close.vi"("error in (no error)"=w544, "connection ID"=w545) -> ("error out"=w543:errorcluster)  [unwired: 1 out]
    }
    frame #1 {
      n231 = call <userlib>:"430_RS232_Close.vi"("error in (no error)"=w548, "VISA resource name"=w546) -> ("error out"=w547:errorcluster)  [unwired: 1 in]
    }
    frame #2 {
    }
  }
  "error out" <- w20
  n232 = local read "Magnetic Field Units"() -> (w47:u16)
  n233 = local read "Coordinate System"() -> (w48:u16)
  n234 = while {
    tunnel: "Starting index" -> [w557]
    tunnel: w22 -> [w563]
    tunnel: w21 -> [w564]
    tunnel: w47 -> [w565]
    tunnel: w48 -> [w566]
    tunnel: w45 -> [w569]
    tunnel: "Max Ramp Rate - Y Axis (A/s)" -> [w553]
    tunnel: "Max Ramp Rate - Z Axis (A/s)" -> [w552]
    tunnel: "Magnitude Limit (kG)" -> [w554]
    tunnel: "User defined Ramp Rate (T/min)" -> [w551]
    tunnel: "User defined Ramp Rate (T/min)" -> [w550]
    i -> [w556]
    stop <- w558 continue-if-true
    n235 = local read "Field Values"() -> (w560:string[][])
    n236 = Add(x=w557, y=w556) -> (x+y=w555:i32)
    n237 = while "Wait for NEXT VECTOR setting by operator." {
      tunnel: [w573] -> w568
      tunnel: w569 -> [w573]
      stop <- w574 continue-if-true
      w572 = u16 0 items=["NEXT VECTOR", "RAMPING", "HOLDING", "PAUSE", "ZERO"] ("Ramping Control")
      n238 = local read "Ramping Control"() -> (w575:u16)
      n239 = Not Equal?(x=w572, y=w575) -> (x != y?=w574:bool)
    }
    n240 = stacked-sequence {
      tunnel: w555 -> [w577 _ w583 _]
      frame #0 {
        (unwired) -2
        n241 = Subtract(x=w577, y=2) -> (x-y=w580:i32)
        n242 = Bundle(w580, -2) -> (w578:cluster{i32, i32})  [unwired: 1 in]
        n243 = property on="Field Values" class="Tbl (strict)"("Active Cell:Active Cell"=w578) -> ()  [unwired: 2 in, 2 out]
      }
      frame #1 {
        n244 = local read "Normal color"() -> (w581:u32)
        n245 = property on="Field Values" class="Tbl (strict)"("Active Cell:Cell Background Color"=w581) -> ()  [unwired: 2 in, 2 out]
      }
      frame #2 {
        n246 = Decrement(x=w583) -> (x-1=w582:i32)
        n247 = Bundle(w582, -2) -> (w585:cluster{i32, i32})  [unwired: 1 in]
        n248 = property on="Field Values" class="Tbl (strict)"("Active Cell:Active Cell"=w585) -> ()  [unwired: 2 in, 2 out]
      }
      frame #3 {
        n249 = property on="Field Values" class="Tbl (strict)"("Active Cell:Cell Background Color"="Highlight color") -> ()  [unwired: 2 in, 2 out]
      }
    }
    n250 = Index Array(array=w560, index (row)=w555) -> (element=w567:string[])  [unwired: 1 in]
    n251 = local write "Starting index"(w555) -> ()
    n252 = Add(x=1, y=w555) -> (x+y=w570:i32)
    n253 = Number To Decimal String(number=w570) -> (decimal integer string=w559:string)  [unwired: 1 in]
    n254 = stacked-sequence {
      tunnel: [_ w611] -> w561
      tunnel: [_ w610] -> w562
      tunnel: w568 -> [_ w606]
      tunnel: w567 -> [_ w605]
      tunnel: w566 -> [_ w604]
      tunnel: w565 -> [_ w603]
      tunnel: w564 -> [_ w602]
      tunnel: w563 -> [_ w601]
      tunnel: w559 -> [_ w600]
      tunnel: w554 -> [_ w598]
      tunnel: w553 -> [_ w597]
      tunnel: w552 -> [_ w592]
      tunnel: w551 -> [_ w596]
      tunnel: w550 -> [_ w595]
      frame #0 {
        w590 = u16 1 items=["NEXT VECTOR", "RAMPING", "HOLDING", "PAUSE", "ZERO"] ("Ramping Control")
        n255 = local write "Ramping Control"(w590) -> ()
      }
      frame #1 {
        n256 = call <userlib>:"Set 2D Next Vector_entwurf.vi"("Coordinate System"=w604, "Magnetic Field Units"=w603, 3:"User defined Ramp Rate (T/min)"=w595, "Magnitude Limit (kG)"=w598, "Y-Axis Communications Config"=w602, "Input Vector"=w605, "Z-Axis Communications Config"=w601, 10:"User defined Ramp Rate (T/min)"=w596, "Max Ramp Rate - Y Axis (A/s)"=w597, "error in"=w606, "Max Ramp Rate - Z Axis (A/s)"=w592) -> ("Y-Axis Ramp Rate (T/min)"=→"Current Ramp Rate Y (T/min)":dbl, "Within Limits?"=w611:bool, "Ramp Rate along Vector (T/min)"=→"Ramp Rate along Vector (T/min)":dbl, "Z-Axis Ramp Rate (T/min)"=→"Current Ramp Rate Z (T/min)":dbl, "All Instruments Responded?"=w610:bool, "error out"=w599:T5)  [unwired: 3 in]
        n257 = Concatenate Strings("Ramping to field vector " ("STATUS"), w600, "..." ("STATUS")) -> (w607:string)
        n258 = local write "error in"(w599) -> ()
        n259 = local write "STATUS"(w607) -> ()
      }
    }
    n260 = case shown="True" w561 {
      tunnel: w562 -> [_ w588]
      frame #0 {
        n261 = local write "STATUS"("Vector magnitude limt or maximum coil current exceeded. Vector ignored. VI halted." ("STATUS")) -> ()
      }
      frame #1 {
        n262 = case shown="True" w588 {
          frame #0 {
            n263 = local write "STATUS"("Not all programmers responded. VI halted." ("STATUS")) -> ()
          }
          frame #1 {
          }
        }
      }
    }
    n264 = Compound Arithmetic op=AND(w562, w561) -> (w558:bool)
    n265 = local write "Continue Execution?"(w558) -> ()
  }
